vi "Ex-1 FPGA soln.vi"() -> ()   [LabVIEW 2014]
uses:
  <vilib>/SPI API/SPIAPI/DIO/SPI Digital IO Lines.ctl
  <vilib>/SPI API/SPIAPI/DIO/SPI DIO Enable Lines.ctl
  <userlib>/_NI SPI IP/FPGA/Controllers/Public/Transfer Settings.ctl
  <vilib>/Platform/TimedLoop/XDataNode/timing_clust.ctl
  <vilib>/Platform/TimedLoop/XDataNode/nitl_modes.ctl
  <vilib>/Platform/TimedLoop/XDataNode/wakeup.ctl
  <vilib>/rvi/Emulation/niFpgaGetClockAttributes.vi
  <vilib>/rvi/Emulation/niFpgaSctlEmulationGetInTimedLoop.vi
  <vilib>/rvi/Emulation/niFpgaEmulationReportErrorSimple.vi
  <vilib>/rvi/Emulation/niFpgaCriticalErrorInLSC.vi
  <vilib>/Platform/TimedLoop/XDataNode/XDataNode.xnode
  <vilib>/Platform/TimedLoop/XDataNode/XDNodeRunTimeDep.lvlib
  <userlib>/_NI SPI IP/FPGA/Controllers/NI SPI IP FPGA.lvlib
panel:
  in  "SPI PHY Settings":T1={"Divide Value"=20, "Transfer Length (bits)"=32, "CS Asserted Polarity"=FALSE, "Clock Polarity (CPOL)"=FALSE, "Clock Phase (CPHA)"=FALSE, "Lengthen MISO Setup"=FALSE, "Direction Change Bit"=0, "MOSI Starts as Output"=FALSE, "Tristatable MOSI"=FALSE} {"Direction Change Bit" max=64 step=1; "Transfer Length (bits)" min=1 max=64 step=1}
  in  "Enable Lines":T2={"SCLK_en"="sbRIO-9651 Socket\\PMOD1_Pin4_enable", "MISO_en"="sbRIO-9651 Socket\\PMOD1_Pin3_enable", "MOSI_en"="sbRIO-9651 Socket\\PMOD1_Pin2_enable", "CS0_en"="sbRIO-9651 Socket\\PMOD1_Pin1_enable", "CS1_en"="sbRIO-9651 Socket\\PMOD1_Pin1_enable", "CS2_en"="sbRIO-9651 Socket\\PMOD1_Pin1_enable", "CS3_en"="sbRIO-9651 Socket\\PMOD1_Pin1_enable", "CS4_en"="sbRIO-9651 Socket\\PMOD1_Pin1_enable", "CS5_en"="sbRIO-9651 Socket\\PMOD1_Pin1_enable"}
  in  "SPI DIO Lines":T3={"SCLK"="sbRIO-9651 Socket\\PMOD1_Pin4_out", "MISO"="sbRIO-9651 Socket\\PMOD1_Pin3_in", "MOSI"="sbRIO-9651 Socket\\PMOD1_Pin2_out", "CS 0"="sbRIO-9651 Socket\\PMOD1_Pin1_out", "CS 1"="sbRIO-9651 Socket\\PMOD1_Pin1_out", "CS 2"="sbRIO-9651 Socket\\PMOD1_Pin1_out", "CS 3"="sbRIO-9651 Socket\\PMOD1_Pin1_out", "CS 4"="sbRIO-9651 Socket\\PMOD1_Pin1_out", "CS 5"="sbRIO-9651 Socket\\PMOD1_Pin1_out"}
  in  "Chip Select":u8
  in  "Data To Device":u64=2147483648 format="%b"
  out "Data from Device":u64(graph)
  # "Put Diagram or Something Here"
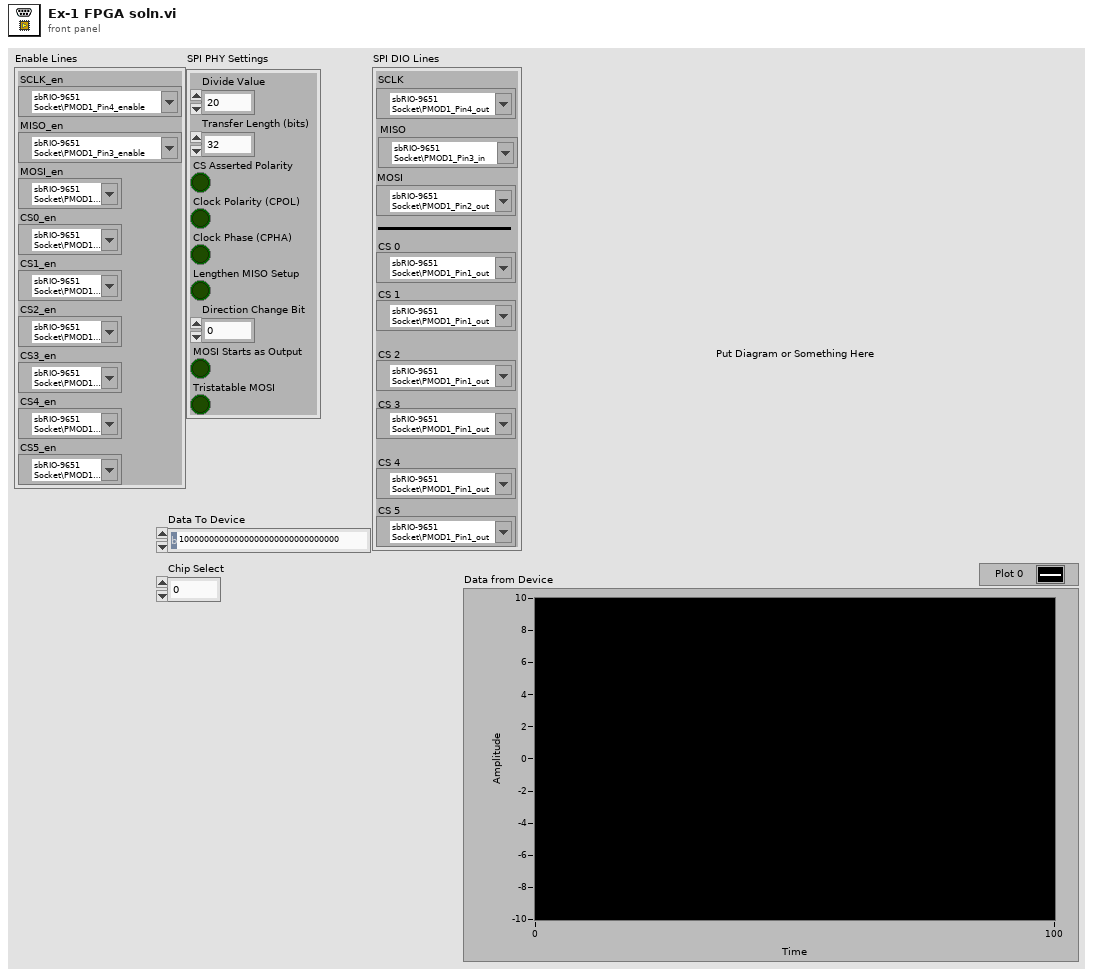
[diagram p1: front panel]
types:
  T1 = typedef "NI SPI IP FPGA.lvlib/Transfer Settings.ctl" = cluster{"Divide Value":u8, "Transfer Length (bits)":u8, "CS Asserted Polarity":bool, "Clock Polarity (CPOL)":bool, "Clock Phase (CPHA)":bool, "Lengthen MISO Setup":bool, "Direction Change Bit":u8, "MOSI Starts as Output":bool, "Tristatable MOSI":bool}
  T2 = typedef "SPI DIO Enable Lines.ctl" = cluster{"SCLK_en":refnum<k21>, "MISO_en":refnum<k21>, "MOSI_en":refnum<k21>, "CS0_en":refnum<k21>, "CS1_en":refnum<k21>, "CS2_en":refnum<k21>, "CS3_en":refnum<k21>, "CS4_en":refnum<k21>, "CS5_en":refnum<k21>}
  T3 = typedef "SPI Digital IO Lines.ctl" = cluster{"SCLK":refnum<k21>, "MISO":refnum<k21>, "MOSI":refnum<k21>, "CS 0":refnum<k21>, "CS 1":refnum<k21>, "CS 2":refnum<k21>, "CS 3":refnum<k21>, "CS 4":refnum<k21>, "CS 5":refnum<k21>}
  T4 = typedef "Internal Data (SPI API).ctl" = cluster{"DLU To SPI Engine Data FIFO":refnum<k21>, "SPI Engine to DLU Data FIFO":refnum<k21>, "Data to SPI Engine (Cache) Register":refnum<k21>, "SPI PHY Settings to SPI Engine (Cahche) Register":refnum<k21>}
  T5 = typedef "XDNodeRunTimeDep.lvlib/timing_clust.ctl" = cluster{"Expected End [f-1]":u64, "Actual End [f-1]":u64, "Finished Late? [f-1]":bool, "Expected End [i-1]":u64, "Actual End [i-1]":u64, "Finished Late? [i-1]":bool, "Expected Start [i]":u64, "Actual Start [i]":u64, "Expected Start [f]":u64, "Actual Start [f]":u64, "Source Name":string, "Structure Name":string, "Period":i64, "Deadline":i64, "Offset":i64, "Start":i64, "Priority":i32, "Timeout":i32, "Mode":T6, "Wakeup Reason":T7, "Error":errorcluster, "Source Type":string, "Secondary Source Type":string, "Global End Time":u64, "Global Start Time":u64, "Frame Duration":u64, "Iteration Duration":u64, "Assigned CPU":i32, "I/O Scan Engine Mode":u32}
  T6 = typedef "XDNodeRunTimeDep.lvlib/nitl_modes.ctl" = enum32{"No Change", "Process missed periods, maintain original phase", "Discard missed periods, maintain original phase", "Process missed periods, ignore original phase", "Discard missed periods, ignore original phase"}
  T7 = typedef "XDNodeRunTimeDep.lvlib/wakeup.ctl" = enum32{"Normal", "Aborted", "Asynchronous wakeup", "Timing source error", "Timed loop error", "Timeout"}
  T8 = typedef "SPI Response Information.ctl" = cluster{"Data to Node":u64, "Node Id":u16}
  T9 = typedef "NI SPI IP FPGA.lvlib/Spi Master Inputs.ctl" = cluster{"MISO":bool}
  T10 = typedef "NI SPI IP FPGA.lvlib/Spi Master Outputs.ctl" = cluster{"Chip Select":bool, "Clock":bool, "MOSI":bool, "MOSI OE":bool}
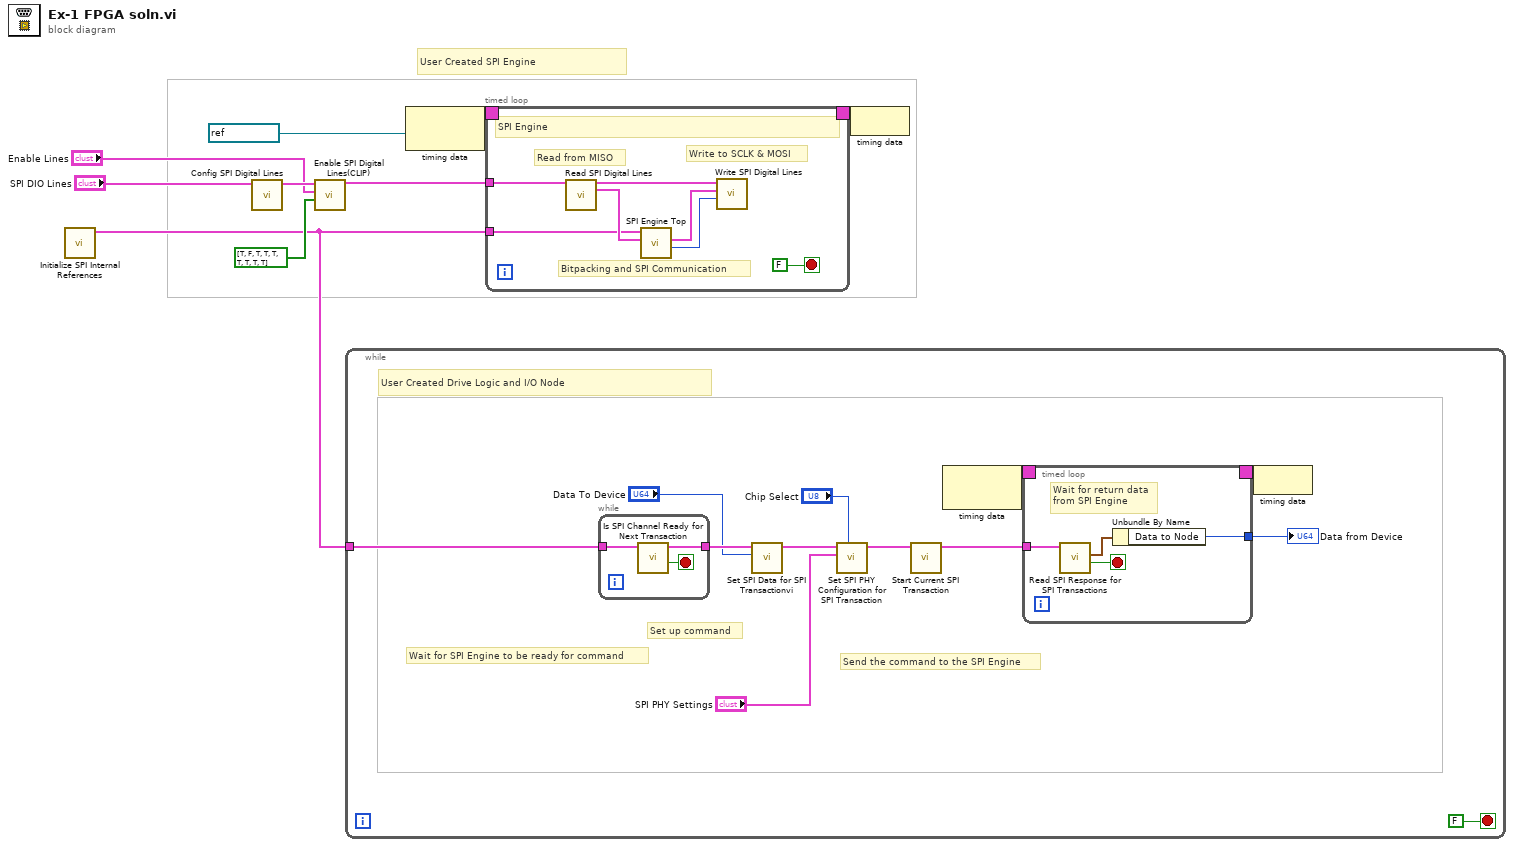
[diagram p0: block diagram]
diagram:
  # "User Created SPI Engine"
  n1 = call <vilib>:"Initialize SPI Internal References.vi"() -> ("SPI API References"=w1:T4)  [unwired: 10 in, 1 out]
  n2 = call <vilib>:"Config SPI Digital Lines.vi"("SPI DIO Lines"="SPI DIO Lines") -> ("Chip Select DIO Lines"=w5:T3)  [unwired: 9 in, 1 out]
  n3 = call <vilib>:"Enable SPI Digital Lines(CLIP).vi"("Enable"=bool[] [TRUE, FALSE, TRUE, TRUE, TRUE, TRUE, TRUE, TRUE, TRUE], "Enable Lines"="Enable Lines", "SPI DIO Lines"=w5) -> ("Chip Select DIO Lines"=w7:T3)  [unwired: 7 in, 1 out]
  n4 = while {
    tunnel: w1 -> [w12]
    stop <- FALSE stop-if-true
    # "Send the command to the SPI Engine"
    # "Set up command"
    # "Wait for SPI Engine to be ready for command"
    # "User Created Drive Logic and I/O Node"
    n5 = while {
      tunnel: w12 -> [w31]
      tunnel: [w30] -> w18
      stop <- w32 stop-if-true
      n6 = call <vilib>:"Is SPI Channel Ready for Next Transaction.vi"("Private Data In"=w31) -> ("SPI Channel Ready"=w32:bool, "Private Data Out"=w30:T4)  [unwired: 7 in, 2 out]
    }
    n7 = call <vilib>:"Set SPI Data for SPI Transactionvi.vi"("Data In"="Data To Device", "Private Data In"=w18) -> ("Private Data Out"=w16:T4)  [unwired: 8 in, 1 out]
    n8 = call <vilib>:"Set SPI PHY Configuration for SPI Transaction.vi"("Chip Select"="Chip Select", "SPI PHY Settings"="SPI PHY Settings", "Private Data In"=w16) -> ("Private Data Out"=w14:T4)  [unwired: 7 in, 1 out]
    n9 = call <vilib>:"Start Current SPI Transaction.vi"("Private Data In"=w14) -> ("Private Data Out"=w13:T4)  [unwired: 8 in, 2 out]
    n10 = node-c288() -> (w21:T5)  [unwired: 1 in]
    n11 = timed-loop {
      timing: w21 -> [_]
      timing-out: [_] -> w20
      tunnel: w13 -> [w25]
      tunnel: [w22] -> w10
      stop <- w24 stop-if-true
      # "Wait for return data\nfrom SPI Engine"
      n12 = call <vilib>:"Read SPI Response for SPI Transactions.vi"("Private Data In"=w25) -> ("Read Data Valid?"=w24:bool, "Read Data"=w23:T8)  [unwired: 7 in, 2 out]
      n13 = Unbundle By Name(w23) -> ("Data to Node"=w22:u64)
    }
    "Data from Device" <- w10
    n14 = node-c288(w20) -> ()
  }
  n15 = node-c288(refnum<k21> "120MHz" ("Source Name")) -> (w9:T5)
  n16 = timed-loop {
    timing: w9 -> [_]
    timing-out: [_] -> w8
    tunnel: w7 -> [w35]
    tunnel: w1 -> [w33]
    stop <- FALSE stop-if-true
    # "Bitpacking and SPI Communication"
    # "Write to SCLK & MOSI"
    # "Read from MISO"
    # "SPI Engine"
    n17 = call <vilib>:"Read SPI Digital Lines.vi"("Chip Select DIO Lines"=w35) -> ("Chip Select DIO Lines Out"=w39:T3, "SPI Read Data"=w38:T9)  [unwired: 12 in, 1 out]
    n18 = call <vilib>:"SPI Engine Top.vi"("SPI Read Data"=w38, "SPI API References"=w33) -> ("Chip Select ID"=w36:u8, "SPI DIO Output"=w37:T10)  [unwired: 6 in, 2 out]
    n19 = call <vilib>:"Write SPI Digital Lines.vi"("CS Index"=w36, "spi output"=w37, "Chip Select DIO Lines"=w39) -> ()  [unwired: 7 in, 2 out]
  }
  n20 = node-c288(w8) -> ()
